vi "시리얼_쓰기.vi"(8 "Error In":errorcluster caption="에러 입력", 10 "Command":string, 11 "VISA 리소스 이름":refnum<visa-resource-name>) -> (0 "Error Out":errorcluster caption="에러 출력", 3 "VISA 리소스 이름 출력":refnum<visa-resource-name>)   [LabVIEW 2015]
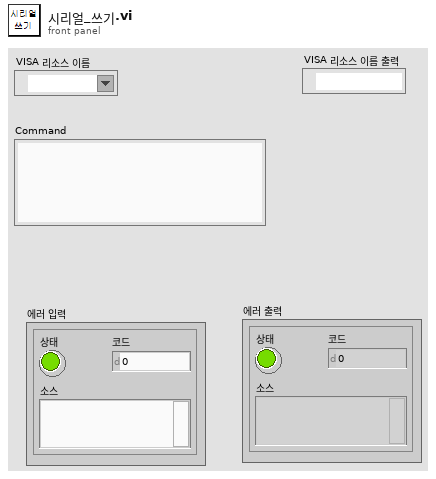
[diagram p1: front panel]
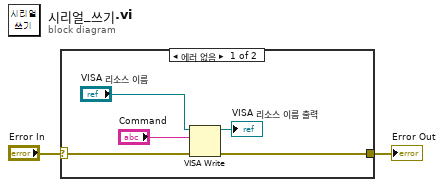
[diagram p0: block diagram]
diagram:
  n1 = case shown="에러 없음" "Error In" {
    selector: "Error In" -> [w7 w8]
    tunnel: [w6 w8] -> w1
    frame No Error {
      n2 = VISA Write(VISA resource name="VISA 리소스 이름", write buffer="Command", error in (no error)=w7) -> (VISA resource name out=→"VISA 리소스 이름 출력":refnum<visa-resource-name>, error out=w6:errorcluster)  [unwired: 1 out]
    }
    frame Error {
    }
  }
  "Error Out" <- w1
